vi "Time_globals.vi"() -> ()   [LabVIEW 2009]
panel:
  out "SP":timestamp
  out "SP-20":timestamp
  out "Start Time":timestamp
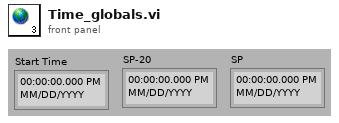
[diagram p1: front panel]
diagram:
